vi "CPL calculator.vi"(8 "GA":dbl=1.0 format="%#_13g", 9 "AGAINx":i32, 10 "ATIME_ms":dbl, 11 "DF":dbl=245.0 format="%#_13g") -> (2 "CPL":dbl)   [LabVIEW 2016, in "AMS TS3472 Light Sensor.lvlib" / "AMS TCS3472.lvclass"]
uses:
  AMS TCS3472.lvclass
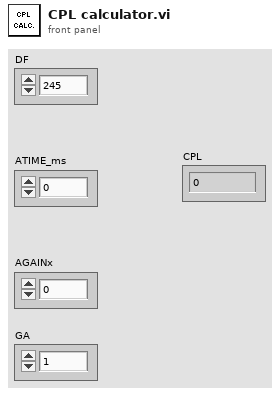
[diagram p1: front panel]
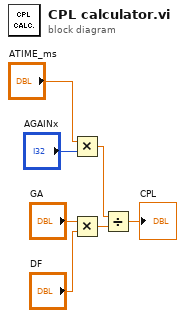
[diagram p0: block diagram]
diagram:
  n1 = Multiply(x="ATIME_ms", y="AGAINx") -> (x*y=w5:dbl)
  n2 = Multiply(x="GA", y="DF") -> (x*y=w2:dbl)
  n3 = Divide(x=w5, y=w2) -> (x/y=→"CPL":dbl)
